vi "Save Image backup2.vi"(8 "Data":dbl[][](array[numeric]), 10 "Process Index":i32, 11 "Current File Num":i32) -> ()   [LabVIEW 2013]
panel:
  out "Path Prefix":string
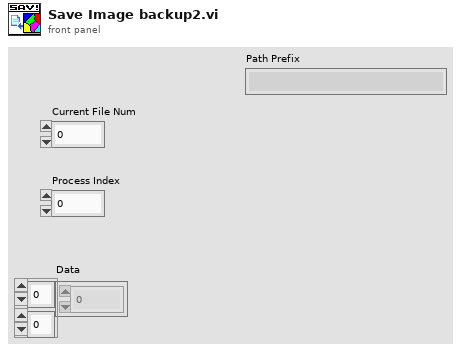
[diagram p1: front panel]
types:
  T1 = typedef "imagedata.ctl" = cluster{"image type":i32, "image depth":i32, "image":u8[], "mask":u8[], "colors":u32[], "Rectangle":cluster{"left":i16, "top":i16, "right":i16, "bottom":i16}}
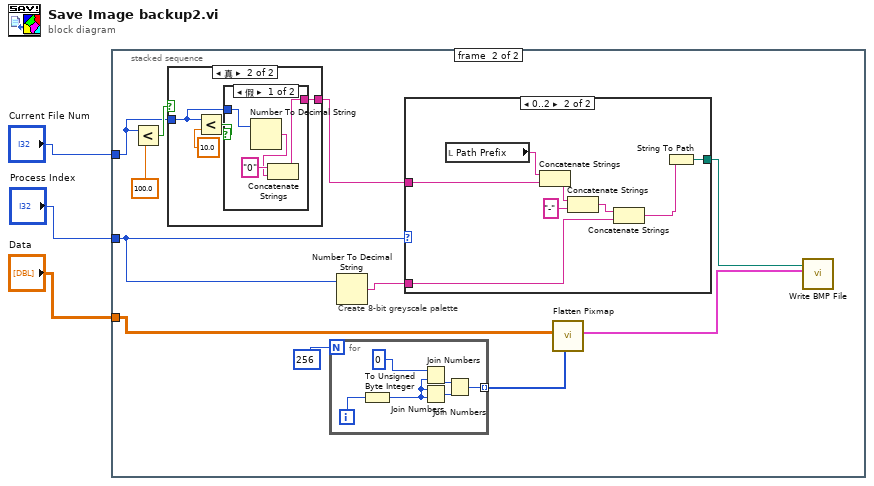
[diagram p0: block diagram]
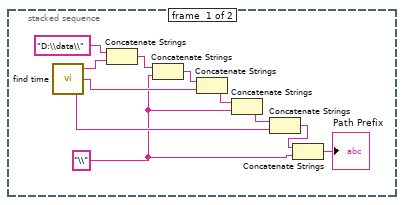
[diagram p2: hidden frame]
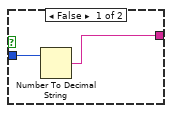
[diagram p3: hidden frame]
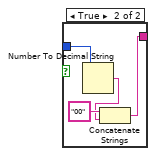
[diagram p4: hidden frame]
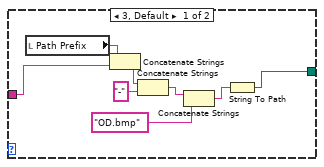
[diagram p5: hidden frame]
diagram:
  n1 = stacked-sequence {
    tunnel: "Current File Num" -> [_ w21]
    tunnel: "Process Index" -> [_ w25]
    tunnel: "Data" -> [_ w18]
    frame #0 {
      w5 = "\\" ("字符串")
      n2 = call "find time.vi"() -> ("day"=w7:string, "month"=w10:string, "year"=w13:string)  [unwired: 3 in]
      n3 = Concatenate Strings("D:\\data\\", w13) -> (w12:string)
      n4 = Concatenate Strings(w12, w5) -> (w11:string)
      n5 = Concatenate Strings(w11, w10) -> (w9:string)
      n6 = Concatenate Strings(w9, w5) -> (w8:string)
      n7 = Concatenate Strings(w8, w7) -> (w6:string)
      n8 = Concatenate Strings(w6, w5) -> (→"Path Prefix":string)
    }
    frame #1 {
      # "Create 8-bit greyscale palette"
      n9 = Less?(x=w21, y=100.0) -> (x < y?=w22:bool)
      n10 = case shown="真" w22 {
        tunnel: w21 -> [w33 w35]
        tunnel: [w32 w34] -> w20
        frame False {
          n11 = Number To Decimal String(number=w33) -> (decimal integer string=w32:string)  [unwired: 1 in]
        }
        frame True {
          n12 = Less?(x=w35, y=10.0) -> (x < y?=w36:bool)
          n13 = case shown="假" w36 {
            tunnel: w35 -> [w40 w45]
            tunnel: [w38 w42] -> w34
            frame False {
              n14 = Number To Decimal String(number=w40) -> (decimal integer string=w39:string)  [unwired: 1 in]
              n15 = Concatenate Strings("0" ("字符串"), w39) -> (w38:string)
            }
            frame True {
              n16 = Number To Decimal String(number=w45) -> (decimal integer string=w43:string)  [unwired: 1 in]
              n17 = Concatenate Strings("00" ("字符串"), w43) -> (w42:string)
            }
          }
        }
      }
      n18 = for {
        N: 256 -> [_]
        tunnel: [w27] -> w17 mode=indexing
        i -> [w29]
        n19 = To Unsigned Byte Integer(number=w29) -> (unsigned 8bit integer=w28:u8)
        n20 = Join Numbers(hi=u8 0, lo=w28) -> ((hi.lo)=w31:u16)
        n21 = Join Numbers(hi=w28, lo=w28) -> ((hi.lo)=w30:u16)
        n22 = Join Numbers(hi=w31, lo=w30) -> ((hi.lo)=w27:u32)
      }
      n23 = Number To Decimal String(number=w25) -> (decimal integer string=w24:string)  [unwired: 1 in]
      n24 = case shown="0..2" w25 {
        tunnel: [w46 w60] -> w16
        tunnel: w20 -> [w49 w59]
        tunnel: w24 -> [_ w55]
        frame 3, Default {
          n25 = local read "Path Prefix"() -> (w50:string)
          n26 = Concatenate Strings(w50, w49) -> (w53:string)
          n27 = Concatenate Strings(w53, "-" ("字符串")) -> (w51:string)
          n28 = Concatenate Strings(w51, "OD.bmp" ("字符串")) -> (w47:string)
          n29 = String To Path(string=w47) -> (path=w46:path)
        }
        frame 0..2 {
          n30 = local read "Path Prefix"() -> (w61:string)
          n31 = Concatenate Strings(w61, w59) -> (w58:string)
          n32 = Concatenate Strings(w58, "-" ("字符串")) -> (w56:string)
          n33 = Concatenate Strings(w56, w55) -> (w54:string)
          n34 = String To Path(string=w54) -> (path=w60:path)
        }
      }
      n35 = call <vilib>:"Flatten Pixmap.vi"("colors"=w17, "8-bit pixmap"=w18) -> ("image data"=w15:T1)  [unwired: 9 in]
      n36 = call <vilib>:"Write BMP File.vi"("image data"=w15, "path to BMP file"=w16) -> ()  [unwired: 8 in, 2 out]
    }
  }
